vi "read pre build action vi.vi"(11 "Builder in":refnum<class "Builder.lvclass">) -> (2 "pre build action vi":path)   [LabVIEW 2024, in "Builder.lvclass"]
uses:
  Builder.lvclass
  Builder.lvclass/Builder.ctl
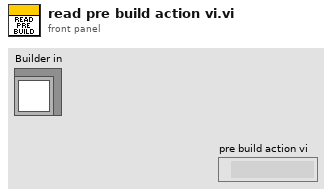
[diagram p1: front panel]
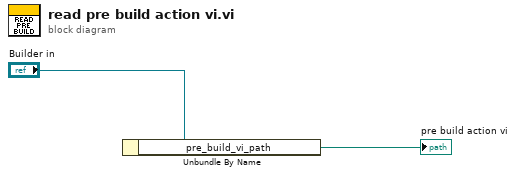
[diagram p0: block diagram]
diagram:
  n1 = Unbundle By Name("Builder in") -> ("pre_build_vi_path"=→"pre build action vi":path)
